vi "Lockin.Low Pass Filter.vi"(8 "error in (no error)":errorcluster, 9 "Y":waveform(dbl)[](array[waveform]), 10 "X":waveform(dbl)[](array[waveform]), 11 "Lockin.DAQ":refnum<class "Instrument.DAQ.lvclass">) -> (0 "error out":errorcluster, 1 "Y out":waveform(dbl)[](array[waveform]), 2 "X out":waveform(dbl)[](array[waveform]), 3 "Lockin.DAQ":refnum<class "Instrument.DAQ.lvclass">)   [LabVIEW 2019, in "Instrument.DAQ.lvclass"]
uses:
  Instrument.DAQ.lvclass
  <userlib>/_OpenG.lib/array/array.llb/Search 1D Array (I32)__ogtk.vi
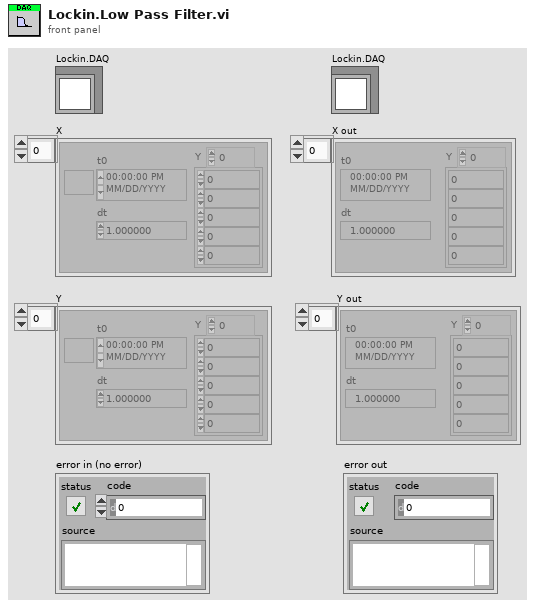
[diagram p1: front panel]
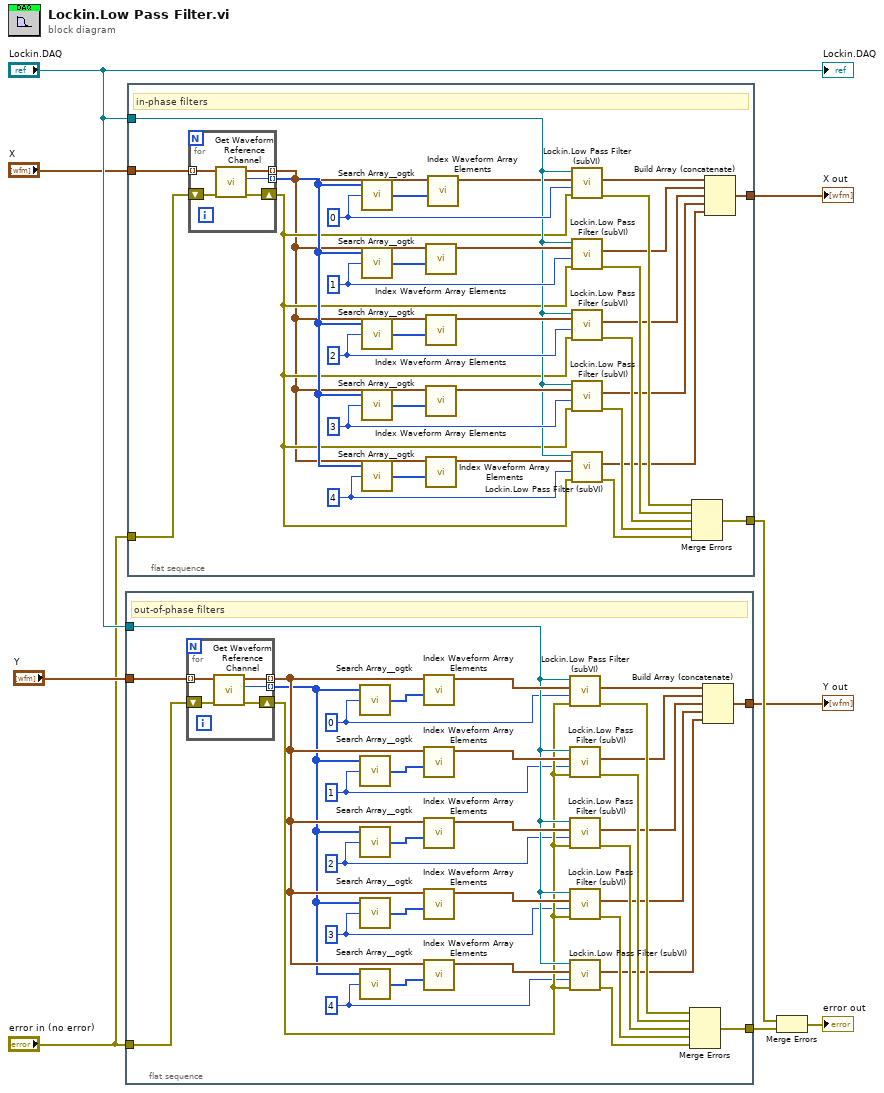
[diagram p0: block diagram]
diagram:
  n1 = flat-sequence {
    tunnel: "error in (no error)" -> [w42]
    tunnel: [w24] -> w7
    tunnel: [w18] -> w3
    tunnel: "Y" -> [w17]
    tunnel: "Lockin.DAQ" -> [w16]
    frame #0 {
      w10 = u16 4 ("Element Data")
      w11 = u16 3 ("Element Data")
      w12 = u16 2 ("Element Data")
      w14 = u16 1 ("Element Data")
      w13 = u16 0 ("Element Data")
      # "out-of-phase filters"
      n2 = for {
        tunnel: [w47] -> w31 mode=indexing
        tunnel: [w46] -> w30 mode=indexing
        tunnel: w17 -> [w45] mode=indexing
        shift-right: [w43] -> w15
        shift-left: w42 -> [w44]
        n3 = call "Get Waveform Reference Channel.vi"("error in (no error)"=w44, "Reference in"=w45) -> ("error out"=w43:errorcluster, "Reference Channel"=w46:i32, "Reference out"=w47:waveform(dbl))  [unwired: 7 in]
      }
      n4 = call-poly <userlib>:"Search Array__ogtk.vi"("Array"=w30, "Element Data"=w13) -> ("Indices of Elements"=w40:i32[])  [unwired: 7 in]
      n5 = call-poly <userlib>:"Search Array__ogtk.vi"("Array"=w30, "Element Data"=w14) -> ("Indices of Elements"=w39:i32[])  [unwired: 7 in]
      n6 = call-poly <userlib>:"Search Array__ogtk.vi"("Array"=w30, "Element Data"=w12) -> ("Indices of Elements"=w36:i32[])  [unwired: 7 in]
      n7 = call-poly <userlib>:"Search Array__ogtk.vi"("Array"=w30, "Element Data"=w11) -> ("Indices of Elements"=w35:i32[])  [unwired: 7 in]
      n8 = call-poly <userlib>:"Search Array__ogtk.vi"("Array"=w30, "Element Data"=w10) -> ("Indices of Elements"=w32:i32[])  [unwired: 7 in]
      n9 = call "Index Waveform Array Elements.vi"("Indices of Elements"=w40, "Array in"=w31) -> ("Array out"=w41:waveform(dbl)[])  [unwired: 9 in]
      n10 = call "Index Waveform Array Elements.vi"("Indices of Elements"=w39, "Array in"=w31) -> ("Array out"=w38:waveform(dbl)[])  [unwired: 9 in]
      n11 = call "Index Waveform Array Elements.vi"("Indices of Elements"=w36, "Array in"=w31) -> ("Array out"=w37:waveform(dbl)[])  [unwired: 9 in]
      n12 = call "Index Waveform Array Elements.vi"("Indices of Elements"=w35, "Array in"=w31) -> ("Array out"=w34:waveform(dbl)[])  [unwired: 9 in]
      n13 = call "Index Waveform Array Elements.vi"("Indices of Elements"=w32, "Array in"=w31) -> ("Array out"=w33:waveform(dbl)[])  [unwired: 9 in]
      n14 = call "Lockin.Low Pass Filter (subVI).vi"("error in (no error)"=w15, "Element Data"=w13, "Array"=w41, "Lockin.DAQ in"=w16) -> ("error out"=w29:errorcluster, "signal out"=w23:waveform(dbl)[])  [unwired: 5 in, 1 out]
      n15 = call "Lockin.Low Pass Filter (subVI).vi"("error in (no error)"=w15, "Element Data"=w14, "Array"=w38, "Lockin.DAQ in"=w16) -> ("error out"=w25:errorcluster, "signal out"=w22:waveform(dbl)[])  [unwired: 5 in, 1 out]
      n16 = call "Lockin.Low Pass Filter (subVI).vi"("error in (no error)"=w15, "Element Data"=w12, "Array"=w37, "Lockin.DAQ in"=w16) -> ("error out"=w26:errorcluster, "signal out"=w21:waveform(dbl)[])  [unwired: 5 in, 1 out]
      n17 = call "Lockin.Low Pass Filter (subVI).vi"("error in (no error)"=w15, "Element Data"=w11, "Array"=w34, "Lockin.DAQ in"=w16) -> ("error out"=w27:errorcluster, "signal out"=w20:waveform(dbl)[])  [unwired: 5 in, 1 out]
      n18 = call "Lockin.Low Pass Filter (subVI).vi"("error in (no error)"=w15, "Element Data"=w10, "Array"=w33, "Lockin.DAQ in"=w16) -> ("error out"=w28:errorcluster, "signal out"=w19:waveform(dbl)[])  [unwired: 5 in, 1 out]
      n19 = Merge Errors(w29, w25, w26, w27, w28) -> (w24:errorcluster)
      n20 = Build Array (concatenate)(w23, w22, w21, w20, w19) -> (w18:waveform(dbl)[])
    }
  }
  n21 = flat-sequence {
    tunnel: "error in (no error)" -> [w80]
    tunnel: [w60] -> w8
    tunnel: [w54] -> w2
    tunnel: "X" -> [w53]
    tunnel: "Lockin.DAQ" -> [w52]
    frame #0 {
      w66 = u16 4 ("Element Data")
      w69 = u16 3 ("Element Data")
      w68 = u16 2 ("Element Data")
      w67 = u16 1 ("Element Data")
      w79 = u16 0 ("Element Data")
      # "in-phase filters"
      n22 = for {
        tunnel: [w85] -> w48 mode=indexing
        tunnel: [w84] -> w70 mode=indexing
        tunnel: w53 -> [w83] mode=indexing
        shift-right: [w81] -> w50
        shift-left: w80 -> [w82]
        n23 = call "Get Waveform Reference Channel.vi"("error in (no error)"=w82, "Reference in"=w83) -> ("error out"=w81:errorcluster, "Reference Channel"=w84:i32, "Reference out"=w85:waveform(dbl))  [unwired: 7 in]
      }
      n24 = call-poly <userlib>:"Search Array__ogtk.vi"("Array"=w70, "Element Data"=w79) -> ("Indices of Elements"=w51:i32[])  [unwired: 7 in]
      n25 = call-poly <userlib>:"Search Array__ogtk.vi"("Array"=w70, "Element Data"=w67) -> ("Indices of Elements"=w78:i32[])  [unwired: 7 in]
      n26 = call-poly <userlib>:"Search Array__ogtk.vi"("Array"=w70, "Element Data"=w68) -> ("Indices of Elements"=w75:i32[])  [unwired: 7 in]
      n27 = call-poly <userlib>:"Search Array__ogtk.vi"("Array"=w70, "Element Data"=w69) -> ("Indices of Elements"=w74:i32[])  [unwired: 7 in]
      n28 = call-poly <userlib>:"Search Array__ogtk.vi"("Array"=w70, "Element Data"=w66) -> ("Indices of Elements"=w71:i32[])  [unwired: 7 in]
      n29 = call "Index Waveform Array Elements.vi"("Indices of Elements"=w78, "Array in"=w48) -> ("Array out"=w77:waveform(dbl)[])  [unwired: 9 in]
      n30 = call "Index Waveform Array Elements.vi"("Indices of Elements"=w75, "Array in"=w48) -> ("Array out"=w76:waveform(dbl)[])  [unwired: 9 in]
      n31 = call "Index Waveform Array Elements.vi"("Indices of Elements"=w74, "Array in"=w48) -> ("Array out"=w73:waveform(dbl)[])  [unwired: 9 in]
      n32 = call "Index Waveform Array Elements.vi"("Indices of Elements"=w71, "Array in"=w48) -> ("Array out"=w72:waveform(dbl)[])  [unwired: 9 in]
      n33 = call "Index Waveform Array Elements.vi"("Indices of Elements"=w51, "Array in"=w48) -> ("Array out"=w49:waveform(dbl)[])  [unwired: 9 in]
      n34 = call "Lockin.Low Pass Filter (subVI).vi"("error in (no error)"=w50, "Element Data"=w79, "Array"=w49, "Lockin.DAQ in"=w52) -> ("error out"=w65:errorcluster, "signal out"=w59:waveform(dbl)[])  [unwired: 5 in, 1 out]
      n35 = call "Lockin.Low Pass Filter (subVI).vi"("error in (no error)"=w50, "Element Data"=w67, "Array"=w77, "Lockin.DAQ in"=w52) -> ("error out"=w61:errorcluster, "signal out"=w58:waveform(dbl)[])  [unwired: 5 in, 1 out]
      n36 = call "Lockin.Low Pass Filter (subVI).vi"("error in (no error)"=w50, "Element Data"=w68, "Array"=w76, "Lockin.DAQ in"=w52) -> ("error out"=w62:errorcluster, "signal out"=w57:waveform(dbl)[])  [unwired: 5 in, 1 out]
      n37 = call "Lockin.Low Pass Filter (subVI).vi"("error in (no error)"=w50, "Element Data"=w69, "Array"=w73, "Lockin.DAQ in"=w52) -> ("error out"=w63:errorcluster, "signal out"=w56:waveform(dbl)[])  [unwired: 5 in, 1 out]
      n38 = call "Lockin.Low Pass Filter (subVI).vi"("error in (no error)"=w50, "Element Data"=w66, "Array"=w72, "Lockin.DAQ in"=w52) -> ("error out"=w64:errorcluster, "signal out"=w55:waveform(dbl)[])  [unwired: 5 in, 1 out]
      n39 = Merge Errors(w65, w61, w62, w63, w64) -> (w60:errorcluster)
      n40 = Build Array (concatenate)(w59, w58, w57, w56, w55) -> (w54:waveform(dbl)[])
    }
  }
  n41 = Merge Errors(w8, w7) -> (→"error out":errorcluster)
  "X out" <- w2
  "Lockin.DAQ" <- "Lockin.DAQ"
  "Y out" <- w3
